vi "Deadzone.vi"(4 "Joystick Livezone":dbl, 5 "Joystick Deadzone":dbl, 8 "Right Joystick":dbl, 9 "Left Joystick":dbl) -> (2 "Right Joystick Refined":dbl, 3 "Left Joystick Refined":dbl)   [LabVIEW 2018]
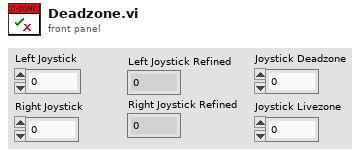
[diagram p1: front panel]
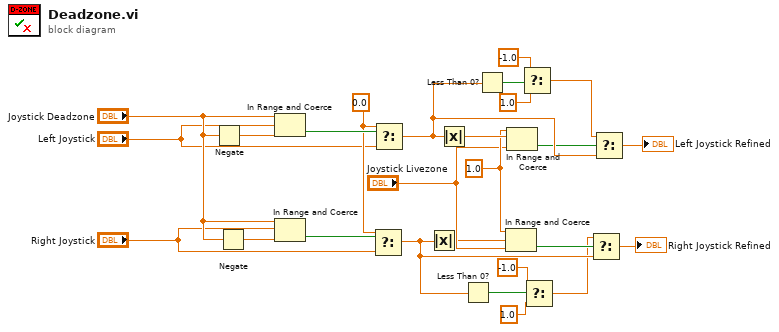
[diagram p0: block diagram]
diagram:
  w11 = 1.0 ("upper limit")
  w21 = 0.0
  n1 = Negate(x="Joystick Deadzone") -> (-x=w26:dbl)
  n2 = Negate(x="Joystick Deadzone") -> (-x=w25:dbl)
  n3 = In Range and Coerce(upper limit="Joystick Deadzone", x="Left Joystick", lower limit=w26) -> (In Range?=w22:bool)  [unwired: 1 out]
  n4 = In Range and Coerce(upper limit="Joystick Deadzone", x="Right Joystick", lower limit=w25) -> (In Range?=w23:bool)  [unwired: 1 out]
  n5 = Select(t=w21, s=w23, f="Right Joystick") -> (s? t:f=w2:dbl)
  n6 = Select(t=w21, s=w22, f="Left Joystick") -> (s? t:f=w13:dbl)
  n7 = Absolute Value(x=w2) -> (abs(x)=w9:dbl)
  n8 = Absolute Value(x=w13) -> (abs(x)=w12:dbl)
  n9 = Less Than 0?(x=w2) -> (x < 0?=w3:bool)
  n10 = Less Than 0?(x=w13) -> (x < 0?=w18:bool)
  n11 = In Range and Coerce(upper limit=w11, x=w9, lower limit="Joystick Livezone") -> (In Range?=w7:bool)  [unwired: 1 out]
  n12 = In Range and Coerce(upper limit=w11, x=w12, lower limit="Joystick Livezone") -> (In Range?=w8:bool)  [unwired: 1 out]
  n13 = Select(t=-1.0, s=w18, f=1.0) -> (s? t:f=w15:dbl)
  n14 = Select(t=-1.0, s=w3, f=1.0) -> (s? t:f=w1:dbl)
  n15 = Select(t=w1, s=w7, f=w2) -> (s? t:f=→"Right Joystick Refined":dbl)
  n16 = Select(t=w15, s=w8, f=w13) -> (s? t:f=→"Left Joystick Refined":dbl)
